vi "Get Image Paths from Folder.vi"(11 "Image Folder":path=path "c:/") -> (3 "Image Paths":path[](array[path]))   [LabVIEW 2016]
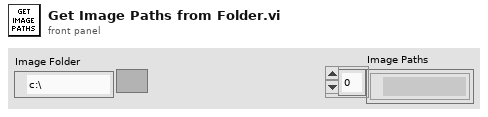
[diagram p1: front panel]
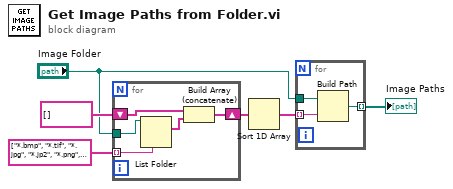
[diagram p0: block diagram]
diagram:
  n1 = for {
    tunnel: "Image Folder" -> [w11]
    shift-right: [w8] -> w5
    shift-left: string[] [] -> [w7]
    tunnel: string[] ["*.bmp", "*.tif", "*.jpg", "*.jp2", "*.png", "*.aipd"] -> [w10] mode=indexing
    n2 = List Folder(path=w11, pattern=w10) -> (filenames=w9:string[])  [unwired: 1 in, 4 out]
    n3 = Build Array (concatenate)(w7, w9) -> (w8:string[])
  }
  n4 = Sort 1D Array(array=w5) -> (sorted array=w2:string[])
  n5 = for {
    tunnel: w2 -> [w14] mode=indexing
    tunnel: "Image Folder" -> [w13]
    tunnel: [w12] -> w1 mode=indexing
    n6 = Build Path(base path=w13, name or relative path=w14) -> (appended path=w12:path)
  }
  "Image Paths" <- w1
